vi "Read Content.vi"(8 "error in (no error)":errorcluster, 11 "Result Table in":refnum<class "Result Table V2.lvclass">) -> (0 "error out":errorcluster, 2 "Result Texts":string[](array[string]), 3 "Result Table out":refnum<class "Result Table V2.lvclass">)   [LabVIEW 2020, in "Result Table V2.lvclass"]
uses:
  Result Table V2.lvclass
  Result Table V2.lvclass/Result Table V2.ctl
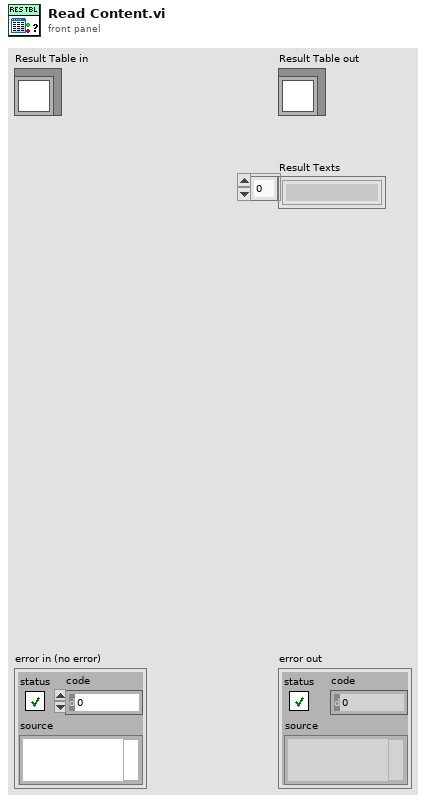
[diagram p1: front panel]
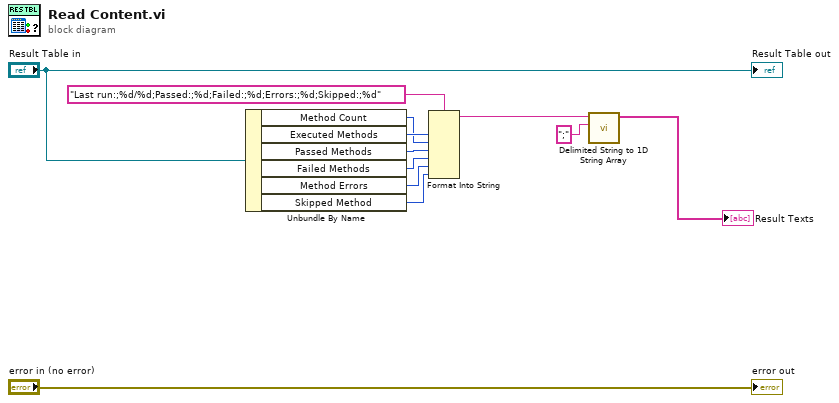
[diagram p0: block diagram]
diagram:
  n1 = Unbundle By Name("Result Table in") -> ("Method Count"=w9:u32, "Executed Methods"=w10:u32, "Passed Methods"=w4:u32, "Failed Methods"=w3:u32, "Method Errors"=w1:u32, "Skipped Method"=w2:u32)
  n2 = Format Into String(format string="Last run:;%d/%d;Passed:;%d;Failed:;%d;Errors:;%d;Skipped:;%d", w10, w9, w4, w3, w1, w2) -> (resulting string=w8:string)  [unwired: 2 in, 1 out]
  n3 = call <vilib>:"Delimited String to 1D String Array.vi"("delimiter"=";", "delimited string"=w8) -> ("string array"=→"Result Texts":string[])  [unwired: 9 in]
  "error out" <- "error in (no error)"
  "Result Table out" <- "Result Table in"
